vi "Balance Data Server.vi"(8 "Time per Block (s)":dbl=100.0 format="%_4f", 11 "Ch No":i16[](array[numeric])) -> (0 "DAQ Error":errorcluster, 2 "Av Sampling Rate":dbl[](array[numeric]), 3 "Time Trace":T1[](array[typedef]))   [LabVIEW 2021]
uses:
  Anemometry/Anemometry Sub Vis/Controls/Time_Trace_Cluster.ctl
  6 Comp Balance Global.vi
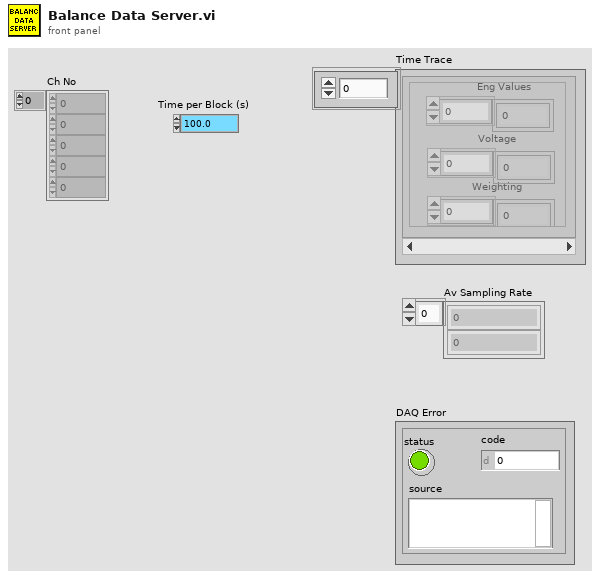
[diagram p1: front panel]
types:
  T1 = typedef "Time_Trace_Cluster.ctl" = cluster{"Weighting":dbl[], "Voltage":dbl[], "Eng Values":dbl[]}
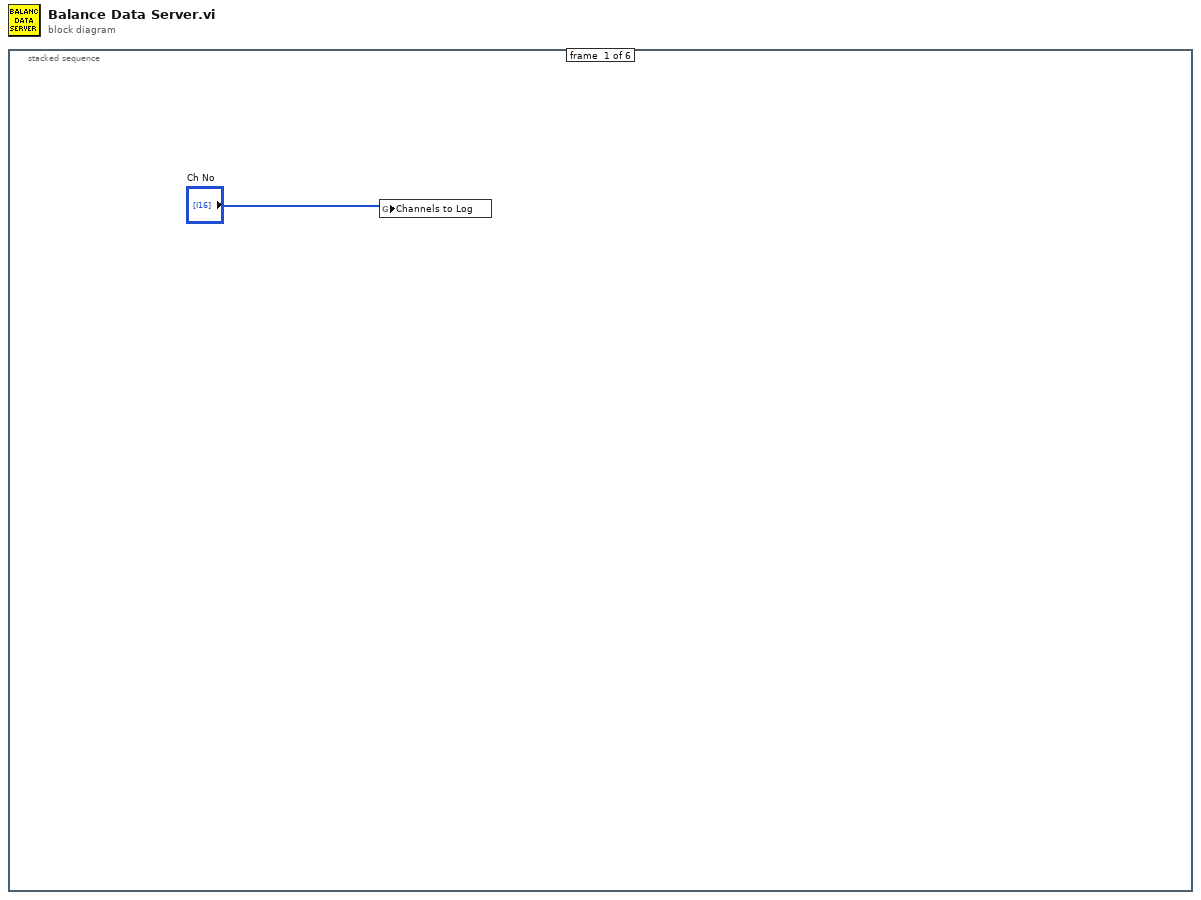
[diagram p0: block diagram]
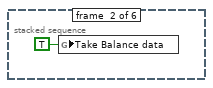
[diagram p2: hidden frame]
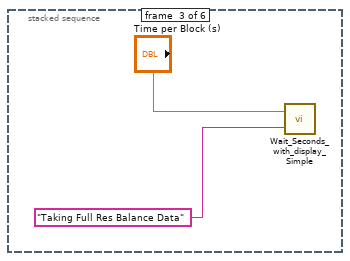
[diagram p3: hidden frame]
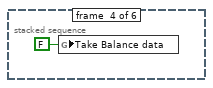
[diagram p4: hidden frame]
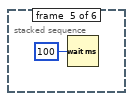
[diagram p5: hidden frame]
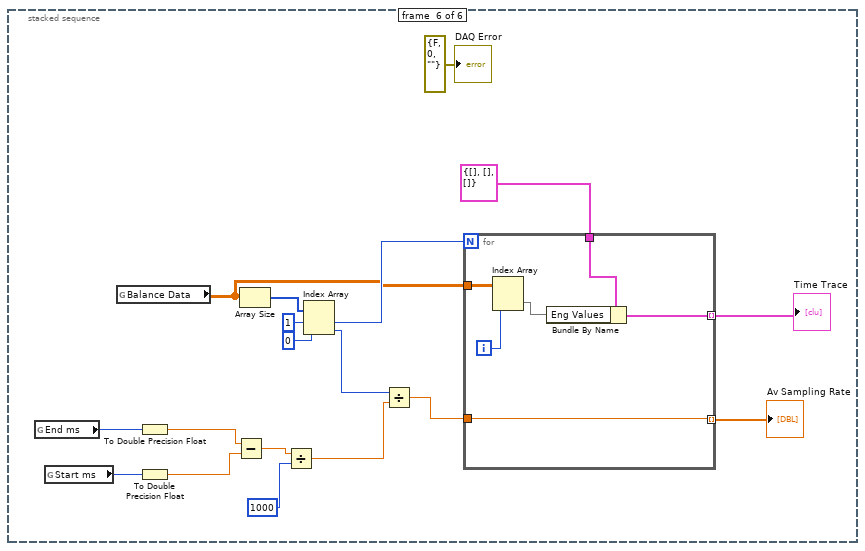
[diagram p6: hidden frame]
diagram:
  n1 = stacked-sequence {
    frame #0 {
      n2 = global write "6 Comp Balance Global.vi" "Channels to Log"("Ch No") -> ()
    }
    frame #1 {
      n3 = global write "6 Comp Balance Global.vi" "Take Balance data"(TRUE ("Take Balance data")) -> ()
    }
    frame #2 {
      n4 = call "Wait_Seconds_with_display_Simple.vi"("Message"="Taking Full Res Balance Data", "Seconds to wait"="Time per Block (s)") -> ()  [unwired: 1 in, 1 out]
    }
    frame #3 {
      n5 = global write "6 Comp Balance Global.vi" "Take Balance data"(FALSE ("Take Balance data")) -> ()
    }
    frame #4 {
      n6 = Wait (ms)(milliseconds to wait=u32 100) -> ()  [unwired: 1 out]
    }
    frame #5 {
      n7 = global read "6 Comp Balance Global.vi" "End ms"() -> (w21:u32)
      n8 = global read "6 Comp Balance Global.vi" "Start ms"() -> (w20:u32)
      n9 = global read "6 Comp Balance Global.vi" "Balance Data"() -> (w12:dbl[][])
      n10 = To Double Precision Float(number=w21) -> (double precision float=w8:dbl)
      n11 = To Double Precision Float(number=w20) -> (double precision float=w7:dbl)
      n12 = Subtract(x=w8, y=w7) -> (x-y=w19:dbl)
      n13 = Array Size(array=w12) -> (size(s)=w22:i32[])
      n14 = Divide(x=w19, y=u32 1000) -> (x/y=w17:dbl)
      n15 = Index Array(array=w22, index #1=1 ("index"), index #2=0 ("index")) -> (element #1=w13:i32, element #2=w14:i32)
      n16 = Divide(x=w14, y=w17) -> (x/y=w16:dbl)
      n17 = for {
        N: w13 -> [_]
        tunnel: [w30] -> w23 mode=indexing
        tunnel: w16 -> [w30]
        tunnel: T1 {"Weighting"=[], "Voltage"=[], "Eng Values"=[]} ("element") -> [w29]
        tunnel: w12 -> [w28]
        tunnel: [w26] -> w11 mode=indexing
        i -> [w25]
        n18 = Index Array(array=w28, index (col)=w25) -> (element=w27:dbl[])  [unwired: 1 in]
        n19 = Bundle By Name(cluster=w29, "Eng Values"=w27) -> (w26:T1)
      }
      "Time Trace" <- w11
      "Av Sampling Rate" <- w23
      "DAQ Error" <- errorcluster {"status"=FALSE, "code"=0, "source"=""} ("DAQ Error")
    }
  }
